vi "读取Allowed VI Alias.vi"(8 "error in (no error)":errorcluster caption="错误输入（无错误）", 11 "PanelDataNode输入":refnum<class "PanelDataNode.lvclass">) -> (0 "error out":errorcluster caption="错误输出", 2 "Allowed VI Alias":string[](array[string]), 3 "PanelDataNode输出":refnum<class "PanelDataNode.lvclass">)   [LabVIEW 2013, in "PanelDataNode.lvclass"]
uses:
  PanelDataNode.lvclass
  PanelDataNode.lvclass/PanelDataNode.ctl
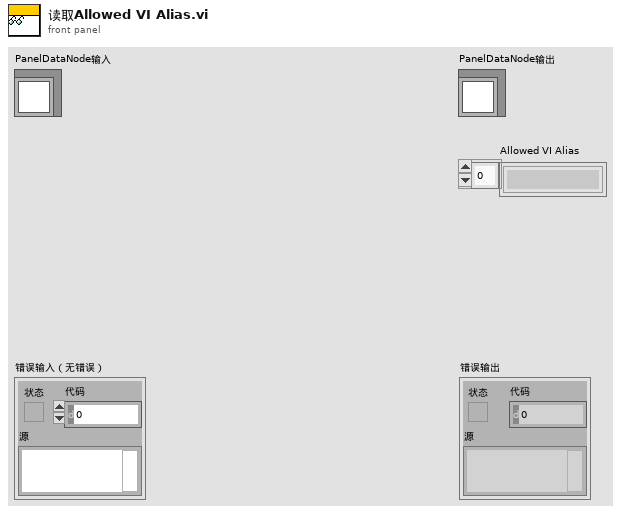
[diagram p1: front panel]
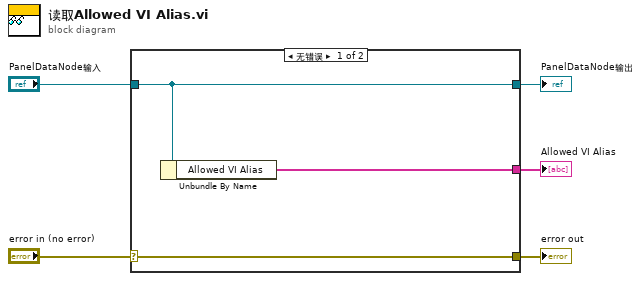
[diagram p0: block diagram]
diagram:
  n1 = case shown="无错误" "error in (no error)" {
    selector: "error in (no error)" -> [w8 w9]
    tunnel: [w8 w9] -> w4
    tunnel: [w7 w10] -> w2
    tunnel: "PanelDataNode输入" -> [w7 w10]
    tunnel: [w6 _] -> w1
    frame No Error {
      n2 = Unbundle By Name(w7) -> ("Allowed VI Alias"=w6:string[])
    }
    frame Error {
    }
  }
  "error out" <- w4
  "PanelDataNode输出" <- w2
  "Allowed VI Alias" <- w1
